vi "Periodic Tasks.vi"(8 "error in":errorcluster) -> ()   [LabVIEW 2016]
doc: "This VI runs in parallel to other tasks. It can contain as many user-defined periodic loops as you need. These can carry out PID or other sorts of timed response."
uses:
  Control 1.ctl
  <vilib>/Rock Robotics/WPI/Solenoid/WPI_SolenoidValue.ctl
  <vilib>/Rock Robotics/WPI/Utilities/WPI_GetSetVariantRefNum.vi
  <vilib>/Rock Robotics/WPI/Solenoid/WPI_SolenoidSetEnum.vi
  <vilib>/Rock Robotics/WPI/Solenoid/WPI_SolenoidGetEnum.vi
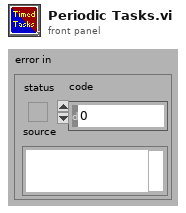
[diagram p1: front panel]
types:
  T1 = typedef "WPI_JoystickDevRef.ctl" = cluster{"Device":T2}
  T2 = typedef "WPI_JoystickDeviceEnum.ctl" = enum16{"USB 0", "USB 1", "USB 2", "USB 3", "USB 4", "USB 5"}
  T3 = typedef "Control 1.ctl" = enum16{"Off", "On"}
  T4 = typedef "WPI_SolenoidValue.ctl" = enum16{"Off", "On", "Forward", "Reverse"}
  T5 = typedef "WPI_SwitchDevRef.ctl" = cluster{"DevStatus":errorcluster, "DIO Channel":T6, "CntIndex":T7, "Normally Closed":bool}
  T6 = typedef "FPGA_DIOChannel.ctl" = enum8{"DIO 0", "DIO 1", "DIO 2", "DIO 3", "DIO 4", "DIO 5", "DIO 6", "DIO 7", "DIO 8", "DIO 9", "DIO MXP 0", "DIO MXP 1", "DIO MXP 2", "DIO MXP 3", "DIO MXP 4", "DIO MXP 5", "DIO MXP 6", "DIO MXP 7", "DIO MXP 8", "DIO MXP 9", "DIO MXP 10", "DIO MXP 11", "DIO MXP 12", "DIO MXP 13", "DIO MXP 14", "DIO MXP 15", "SPI Port CS1", "SPI Port CS2", "SPI Port CS3", "SPI Port MISO", "SPI Port MOSI", "Invalid"}
  T7 = typedef "FPGA_CounterCtrSystemIndex.ctl" = enum8{"Ctr 0", "Ctr 1", "Ctr 2", "Ctr 3", "Ctr 4", "Ctr 5", "Ctr 6", "Ctr 7", "Invalid"}
  T8 = typedef "WPI_SolenoidDevRef.ctl" = cluster{"DevStatus":errorcluster, "Pneumatics Control Module":u8, "Forward Solenoid Channel":T9, "Reverse Solenoid Channel":T9}
  T9 = typedef "WPI_SolenoidChannel.ctl" = enum8{"Solenoid 0", "Solenoid 1", "Solenoid 2", "Solenoid 3", "Solenoid 4", "Solenoid 5", "Solenoid 6", "Solenoid 7", "Invalid"}
  T10 = typedef "WPI_RelayDevRef.ctl" = cluster{"DevStatus":errorcluster, "Relay Channel":T11, "Relay Direction":T12}
  T11 = typedef "FPGA_DIORelayChannel.ctl" = enum8{"Relay 0", "Relay 1", "Relay 2", "Relay 3", "Invalid"}
  T12 = typedef "WPI_RelayDirection.ctl" = enum16{"Both directions", "Forward only", "Reverse only"}
  T13 = typedef "WPI_MotorControlDeviceRef.ctl" = cluster{"DeviceStatus":errorcluster, "Type":T14, "PWM":cluster{"PWM Channel":T15, "DeadBand":T16}, "CAN":cluster{"Device Number":u8, "SetOutput VI Ref":variant, "GetOutput VI Ref":variant, "Enable VI Ref":variant, "Disable VI Ref":variant, "Data":variant}, "Invert":bool}
  T14 = typedef "WPI_MotorControlType.ctl" = enum16{"PWM", "CAN"}
  T15 = typedef "FPGA_DIOPWMChannel.ctl" = enum8{"PWM 0", "PWM 1", "PWM 2", "PWM 3", "PWM 4", "PWM 5", "PWM 6", "PWM 7", "PWM 8", "PWM 9", "PWM MXP 0", "PWM MXP 1", "PWM MXP 2", "PWM MXP 3", "PWM MXP 4", "PWM MXP 5", "PWM MXP 6", "PWM MXP 7", "PWM MXP 8", "PWM MXP 9", "Invalid"}
  T16 = typedef "WPI_PWMDeadband.ctl" = cluster{"Name":string, "maxPositivePwm":i32, "minPositivePwm":i32, "centerPwm":i32, "maxNegativePwm":i32, "minNegativePwm":i32, "angularRange":u16}
  T17 = typedef "WPI_RobotDriveDevRef.ctl" = cluster{"DevStatus":errorcluster, "Motors[]":T13[], "Square Inputs":bool, "Max Output":dbl}
  T18 = cluster{"JoystickDevRef":T1, "JoystickDevRef":T1, "RobotDriveDevRef":T17}
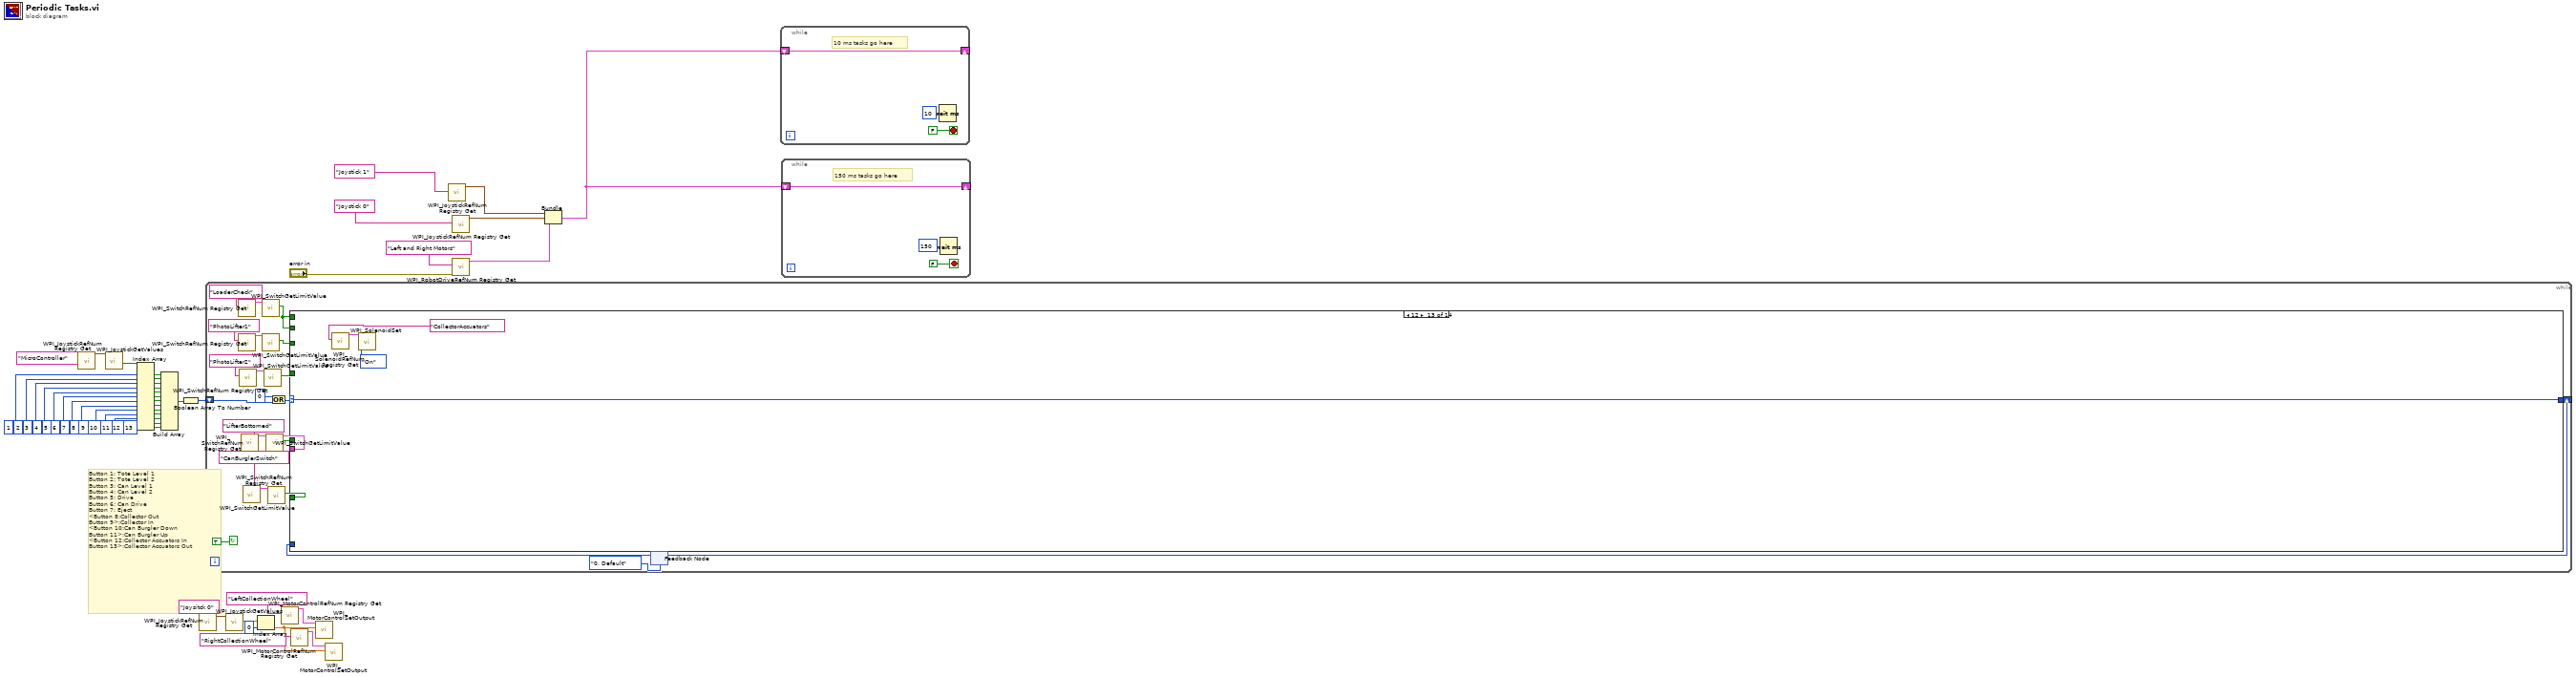
[diagram p0: block diagram]
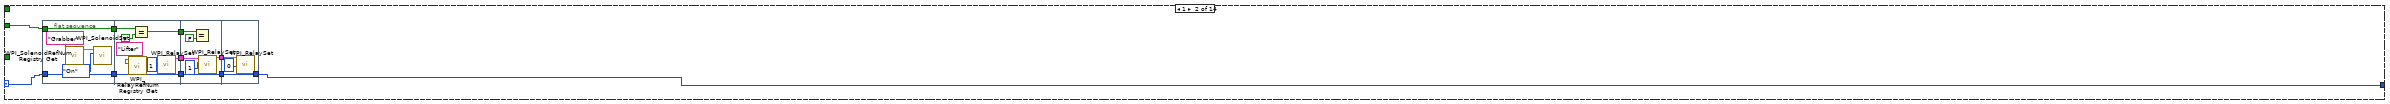
[diagram p3: hidden frame]
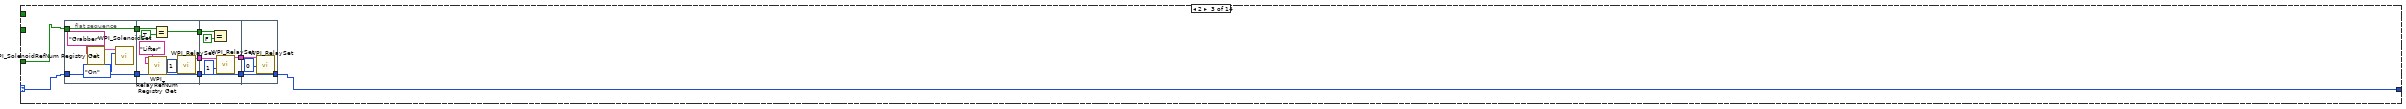
[diagram p4: hidden frame]
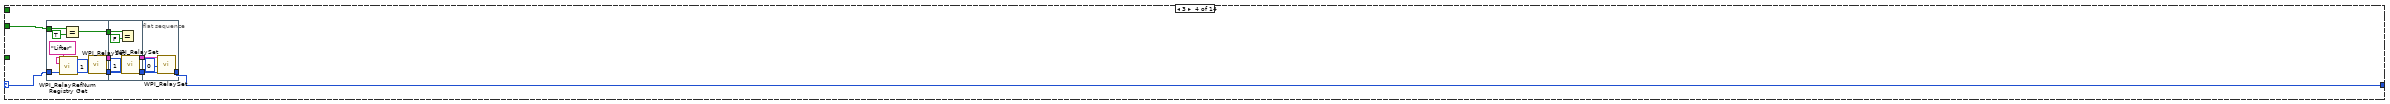
[diagram p5: hidden frame]
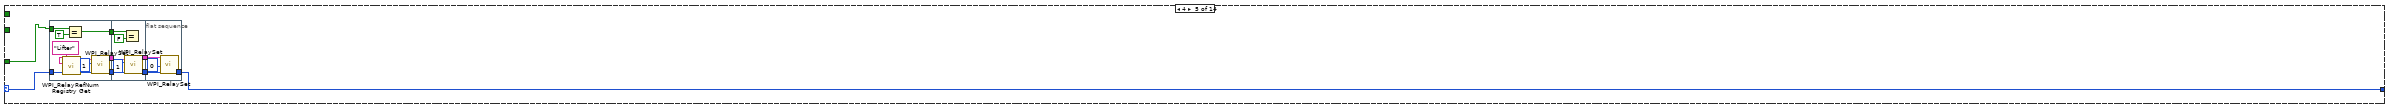
[diagram p6: hidden frame]
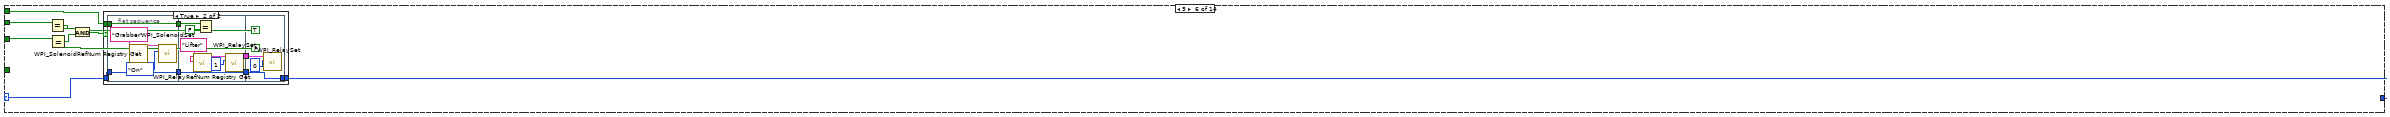
[diagram p7: hidden frame]
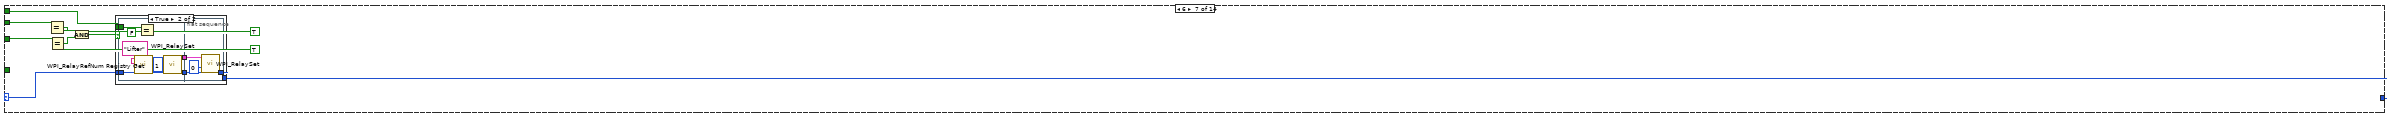
[diagram p9: hidden frame]
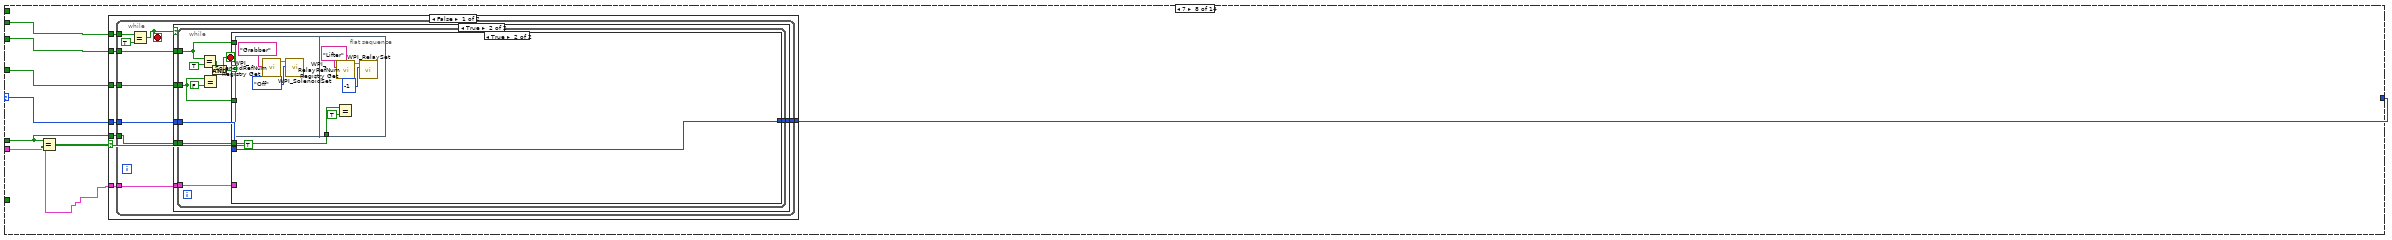
[diagram p11: hidden frame]
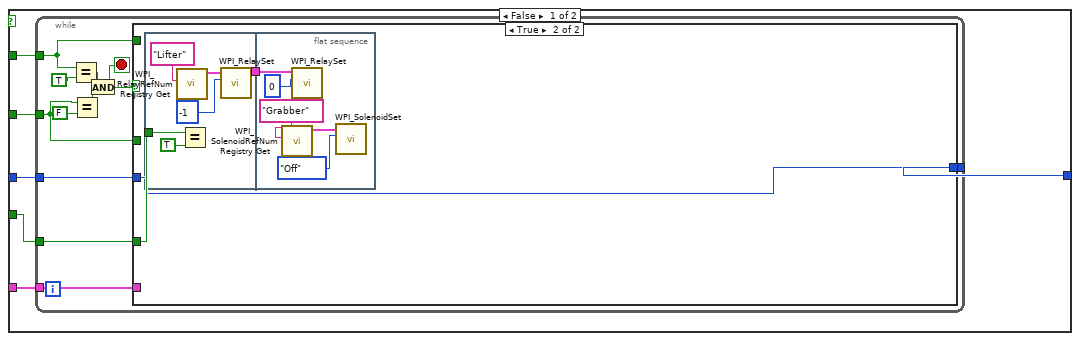
[diagram p12: hidden frame]
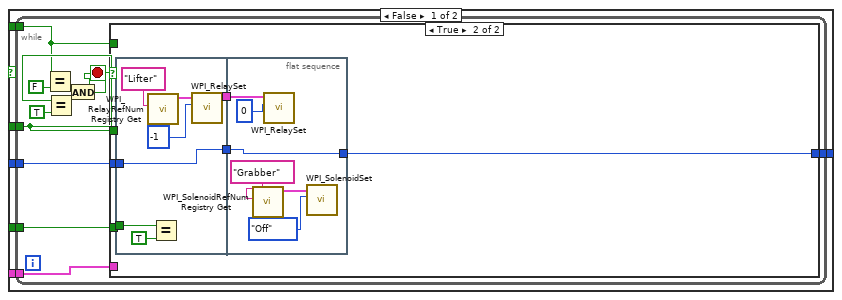
[diagram p13: hidden frame]
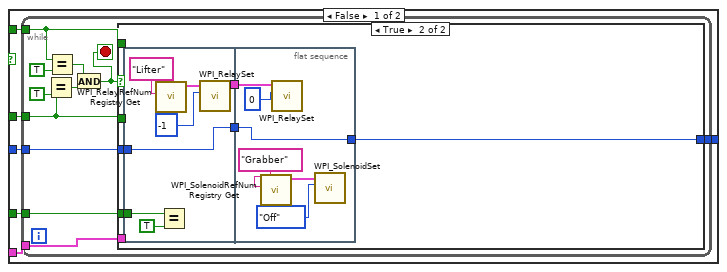
[diagram p14: hidden frame]
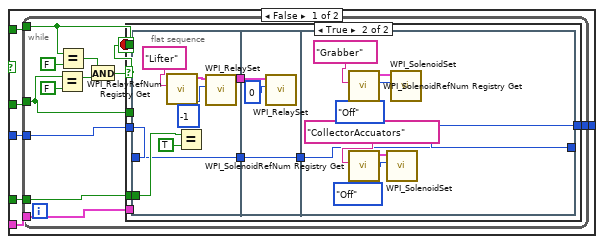
[diagram p15: hidden frame]
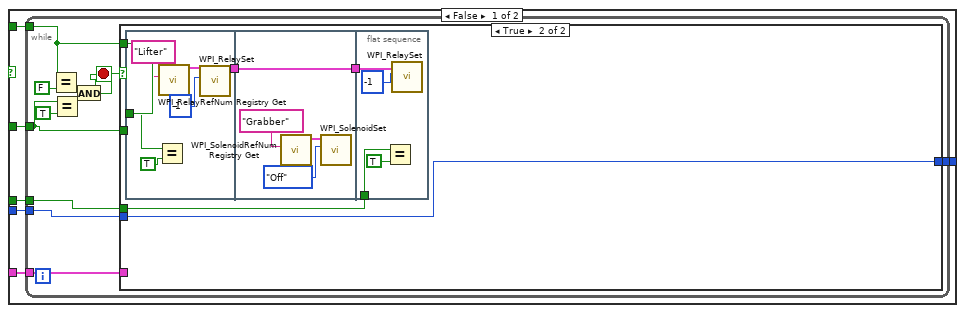
[diagram p17: hidden frame]
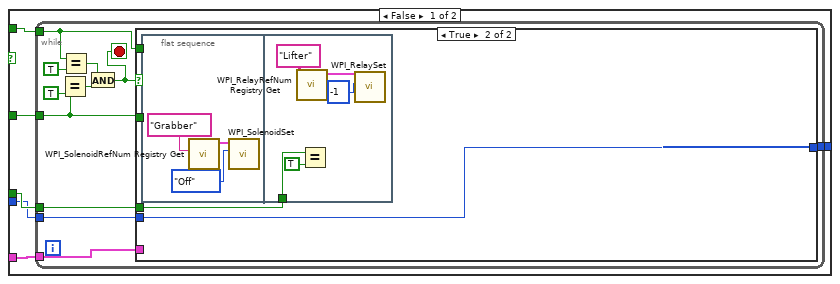
[diagram p18: hidden frame]
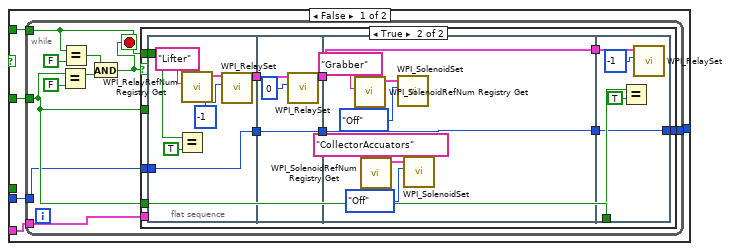
[diagram p19: hidden frame]
diagram:
  # "Button 1: Tote Level 1\nButton 2: Tote Level 2\nButton 3: Can Level 1\nButton 4: Can Level 2\nButton 5: Drive\nButton 6: Can Drive\nButton 7: Eject\n<Button 8:Collector Out\nButton 9>:Collector In\n<Button 10:Can Burgler Down\nButton 11>:Can Burgler Up\n<Button 12:Collector Accuators In\nButton 13>:Collector Accuators Out"
  n1 = call <vilib>:"WPI_JoystickRefNum Registry Get.vi"("refnum name"="MicroController") -> ("JoystickDevRef"=w40:T1)  [unwired: 9 in, 1 out]
  n2 = call <vilib>:"WPI_JoystickGetValues.vi"("JoystickDevRef"=w40) -> ("Buttons"=w39:bool[])  [unwired: 6 in, 4 out]
  n3 = Index Array(array=w39, index #1=1, index #2=2, index #3=3, index #4=4, index #5=5, index #6=6, index #7=7, index #8=8, index #9=9, index #10=10, index #11=11, index #12=12, index #13=13) -> (element #1=w25:bool, element #2=w24:bool, element #3=w23:bool, element #4=w22:bool, element #5=w21:bool, element #6=w20:bool, element #7=w19:bool, element #8=w18:bool, element #9=w17:bool, element #10=w16:bool, element #11=w15:bool, element #12=w14:bool, element #13=w13:bool)
  n4 = Build Array(w25, w24, w23, w22, w21, w20, w19, w18, w17, w16, w15, w14, w13) -> (w12:bool[])
  n5 = Boolean Array To Number(Boolean array=w12) -> (number=w11:u32)
  n6 = call <vilib>:"WPI_JoystickRefNum Registry Get.vi"("refnum name"="Joysitck 0") -> ("JoystickDevRef"=w9:T1)  [unwired: 9 in, 1 out]
  n7 = while {
    shift-right: [w58] -> _
    shift-left: w11 -> [w62]
    stop <- TRUE continue-if-true
    n8 = call <vilib>:"WPI_SwitchRefNum Registry Get.vi"("refnum name"="LoaderCheck") -> ("SwitchDevRef"=w65:T5)  [unwired: 9 in, 1 out]
    n9 = call <vilib>:"WPI_SwitchRefNum Registry Get.vi"("refnum name"="PhotoLifter1") -> ("SwitchDevRef"=w71:T5)  [unwired: 9 in, 1 out]
    n10 = call <vilib>:"WPI_SwitchRefNum Registry Get.vi"("refnum name"="PhotoLifter2") -> ("SwitchDevRef"=w70:T5)  [unwired: 9 in, 1 out]
    n11 = call <vilib>:"WPI_SwitchRefNum Registry Get.vi"("refnum name"="LifterBottomed") -> ("SwitchDevRef"=w55:T5)  [unwired: 9 in, 1 out]
    n12 = call <vilib>:"WPI_SwitchRefNum Registry Get.vi"("refnum name"="CanBurglerSwitch") -> ("SwitchDevRef"=w51:T5)  [unwired: 9 in, 1 out]
    n13 = call <vilib>:"WPI_SwitchGetLimitValue.vi"("SwitchDevRef"=w65) -> ("Switch Pressed"=w63:bool)  [unwired: 8 in, 2 out]
    n14 = call <vilib>:"WPI_SwitchGetLimitValue.vi"("SwitchDevRef"=w71) -> ("Switch Pressed"=w67:bool)  [unwired: 8 in, 2 out]
    n15 = call <vilib>:"WPI_SwitchGetLimitValue.vi"("SwitchDevRef"=w70) -> ("Switch Pressed"=w66:bool)  [unwired: 8 in, 2 out]
    n16 = call <vilib>:"WPI_SwitchGetLimitValue.vi"("SwitchDevRef"=w55) -> ("Switch Pressed"=w54:bool, "SwitchDevRef"=w52:T5)  [unwired: 8 in, 1 out]
    n17 = call <vilib>:"WPI_SwitchGetLimitValue.vi"("SwitchDevRef"=w51) -> ("Switch Pressed"=w49:bool)  [unwired: 8 in, 2 out]
    n18 = Or(x=0, y=w62) -> (x .or. y?=w60:u32)
    n19 = feedback #1(enum16{"0, Default"}."0, Default") -> (w57:u32)
    n20 = case shown="12" w60 {
      selector: w60 -> [w72 w76 w106 w138 w163 w189 w221 w247 w572 w580 _ _ w622 w626]
      tunnel: w67 -> [_ w82 _ w139 _ w196 w225 w251 _ _ _ _ _ _]
      tunnel: [w72 w75 w105 w137 w162 w187 w220 w246 w572 w579 _ _ w622 w626] -> w58
      tunnel: w66 -> [_ _ w107 _ w164 _ _ w250 _ _ _ _ _ _]
      tunnel: w63 -> [_ _ _ _ _ w194 w226 w252 _ w581 _ _ _ _]
      tunnel: w63 -> [_ _ _ _ _ w188 w222 _ _ _ _ _ _ _]
      tunnel: w57 -> [_ _ _ _ _ _ _ _ _ _ _ _ _ _]
      tunnel: w54 -> [_ _ _ _ _ _ _ w248 _ _ _ _ _ _]
      tunnel: w52 -> [_ _ _ _ _ _ _ w249 _ _ _ _ _ _]
      tunnel: w49 -> [_ _ _ _ _ _ _ _ _ _ _ w615 _ _]
      frame 0, Default {
      }
      frame 1 {
        n21 = flat-sequence {
          tunnel: w76 -> [w86]
          tunnel: w82 -> [w87]
          tunnel: [w87] -> w74
          tunnel: [w86] -> w73
          tunnel: [w90] -> w81
          tunnel: [w89] -> w80
          tunnel: [w88] -> w77
          tunnel: w74 -> [w93]
          tunnel: w73 -> [w88]
          tunnel: w81 -> [w101]
          tunnel: w80 -> [w99]
          tunnel: [w97] -> w79
          tunnel: [w96] -> w78
          tunnel: w77 -> [w96]
          tunnel: w79 -> [w104]
          tunnel: [w102] -> w75
          tunnel: w78 -> [w102]
          frame #0 {
            n22 = call <vilib>:"WPI_SolenoidRefNum Registry Get.vi"("refnum name"="Grabber") -> ("SolenoidDevRef"=w85:T8)  [unwired: 9 in, 1 out]
            n23 = call-poly <vilib>:"WPI_SolenoidSet.vi"("Value"=enum16{"Off", "On"}."On", "SolenoidDevRef"=w85) -> ()  [unwired: 8 in, 2 out]
          }
          frame #1 {
            n24 = call <vilib>:"WPI_RelayRefNum Registry Get.vi"("refnum name"="Lifter") -> ("RelayDevRef"=w95:T10)  [unwired: 9 in, 1 out]
            n25 = Equal?(x=w93, y=TRUE) -> (x = y?=w90:bool)
            n26 = call <vilib>:"WPI_RelaySet.vi"("RelayValue"=1, "RelayDevRef"=w95) -> ("RelayDevRef"=w89:T10)  [unwired: 8 in, 1 out]
          }
          frame #2 {
            n27 = Equal?(x=w101, y=FALSE) -> ()  [unwired: 1 out]
            n28 = call <vilib>:"WPI_RelaySet.vi"("RelayValue"=1, "RelayDevRef"=w99) -> ("RelayDevRef"=w97:T10)  [unwired: 8 in, 1 out]
          }
          frame #3 {
            n29 = call <vilib>:"WPI_RelaySet.vi"("RelayValue"=0, "RelayDevRef"=w104) -> ()  [unwired: 8 in, 2 out]
          }
        }
      }
      frame 2 {
        n30 = flat-sequence {
          tunnel: w106 -> [w118]
          tunnel: w107 -> [w119]
          tunnel: [w119] -> w114
          tunnel: [w118] -> w113
          tunnel: [w122] -> w112
          tunnel: [w121] -> w111
          tunnel: [w120] -> w110
          tunnel: w114 -> [w125]
          tunnel: w113 -> [w120]
          tunnel: w112 -> [w133]
          tunnel: w111 -> [w131]
          tunnel: [w129] -> w109
          tunnel: [w128] -> w108
          tunnel: w110 -> [w128]
          tunnel: w109 -> [w136]
          tunnel: [w134] -> w105
          tunnel: w108 -> [w134]
          frame #0 {
            n31 = call <vilib>:"WPI_SolenoidRefNum Registry Get.vi"("refnum name"="Grabber") -> ("SolenoidDevRef"=w117:T8)  [unwired: 9 in, 1 out]
            n32 = call-poly <vilib>:"WPI_SolenoidSet.vi"("Value"=enum16{"Off", "On"}."On", "SolenoidDevRef"=w117) -> ()  [unwired: 8 in, 2 out]
          }
          frame #1 {
            n33 = call <vilib>:"WPI_RelayRefNum Registry Get.vi"("refnum name"="Lifter") -> ("RelayDevRef"=w127:T10)  [unwired: 9 in, 1 out]
            n34 = Equal?(x=w125, y=TRUE) -> (x = y?=w122:bool)
            n35 = call <vilib>:"WPI_RelaySet.vi"("RelayValue"=1, "RelayDevRef"=w127) -> ("RelayDevRef"=w121:T10)  [unwired: 8 in, 1 out]
          }
          frame #2 {
            n36 = Equal?(x=w133, y=FALSE) -> ()  [unwired: 1 out]
            n37 = call <vilib>:"WPI_RelaySet.vi"("RelayValue"=1, "RelayDevRef"=w131) -> ("RelayDevRef"=w129:T10)  [unwired: 8 in, 1 out]
          }
          frame #3 {
            n38 = call <vilib>:"WPI_RelaySet.vi"("RelayValue"=0, "RelayDevRef"=w136) -> ()  [unwired: 8 in, 2 out]
          }
        }
      }
      frame 3 {
        n39 = flat-sequence {
          tunnel: [w147] -> w144
          tunnel: [w146] -> w143
          tunnel: [w145] -> w142
          tunnel: w139 -> [w150]
          tunnel: w138 -> [w145]
          tunnel: w144 -> [w158]
          tunnel: w143 -> [w156]
          tunnel: [w154] -> w141
          tunnel: [w153] -> w140
          tunnel: w142 -> [w153]
          tunnel: w141 -> [w161]
          tunnel: [w159] -> w137
          tunnel: w140 -> [w159]
          frame #0 {
            n40 = call <vilib>:"WPI_RelayRefNum Registry Get.vi"("refnum name"="Lifter") -> ("RelayDevRef"=w152:T10)  [unwired: 9 in, 1 out]
            n41 = Equal?(x=w150, y=TRUE) -> (x = y?=w147:bool)
            n42 = call <vilib>:"WPI_RelaySet.vi"("RelayValue"=1, "RelayDevRef"=w152) -> ("RelayDevRef"=w146:T10)  [unwired: 8 in, 1 out]
          }
          frame #1 {
            n43 = Equal?(x=w158, y=FALSE) -> ()  [unwired: 1 out]
            n44 = call <vilib>:"WPI_RelaySet.vi"("RelayValue"=1, "RelayDevRef"=w156) -> ("RelayDevRef"=w154:T10)  [unwired: 8 in, 1 out]
          }
          frame #2 {
            n45 = call <vilib>:"WPI_RelaySet.vi"("RelayValue"=0, "RelayDevRef"=w161) -> ()  [unwired: 8 in, 2 out]
          }
        }
      }
      frame 4 {
        n46 = flat-sequence {
          tunnel: [w172] -> w169
          tunnel: [w171] -> w168
          tunnel: [w170] -> w167
          tunnel: w164 -> [w175]
          tunnel: w163 -> [w170]
          tunnel: w169 -> [w183]
          tunnel: w168 -> [w181]
          tunnel: [w179] -> w166
          tunnel: [w178] -> w165
          tunnel: w167 -> [w178]
          tunnel: w166 -> [w186]
          tunnel: [w184] -> w162
          tunnel: w165 -> [w184]
          frame #0 {
            n47 = call <vilib>:"WPI_RelayRefNum Registry Get.vi"("refnum name"="Lifter") -> ("RelayDevRef"=w177:T10)  [unwired: 9 in, 1 out]
            n48 = Equal?(x=w175, y=TRUE) -> (x = y?=w172:bool)
            n49 = call <vilib>:"WPI_RelaySet.vi"("RelayValue"=1, "RelayDevRef"=w177) -> ("RelayDevRef"=w171:T10)  [unwired: 8 in, 1 out]
          }
          frame #1 {
            n50 = Equal?(x=w183, y=FALSE) -> ()  [unwired: 1 out]
            n51 = call <vilib>:"WPI_RelaySet.vi"("RelayValue"=1, "RelayDevRef"=w181) -> ("RelayDevRef"=w179:T10)  [unwired: 8 in, 1 out]
          }
          frame #2 {
            n52 = call <vilib>:"WPI_RelaySet.vi"("RelayValue"=0, "RelayDevRef"=w186) -> ()  [unwired: 8 in, 2 out]
          }
        }
      }
      frame 5 {
        n53 = Equal?(x=w194, y=TRUE) -> (x = y?=w192:bool)
        n54 = Equal?(x=w196, y=FALSE) -> (x = y?=w191:bool)
        n55 = And(x=w192, y=w191) -> (x .and. y?=w190:bool)
        n56 = case shown="True" w190 {
          tunnel: w189 -> [w197 w200]
          tunnel: w188 -> [_ w199]
          tunnel: [w197 w198] -> w187
          frame False {
          }
          frame True {
            n57 = flat-sequence {
              tunnel: w200 -> [w208]
              tunnel: w199 -> [w209]
              tunnel: [w209] -> w204
              tunnel: [w208] -> w203
              tunnel: [w211] -> w202
              tunnel: [w210] -> w201
              tunnel: w204 -> [w214]
              tunnel: w203 -> [w210]
              tunnel: w202 -> [w219]
              tunnel: w201 -> [w217]
              tunnel: [w217] -> w198
              frame #0 {
                n58 = call <vilib>:"WPI_SolenoidRefNum Registry Get.vi"("refnum name"="Grabber") -> ("SolenoidDevRef"=w207:T8)  [unwired: 9 in, 1 out]
                n59 = call-poly <vilib>:"WPI_SolenoidSet.vi"("Value"=enum16{"Off", "On"}."On", "SolenoidDevRef"=w207) -> ()  [unwired: 8 in, 2 out]
              }
              frame #1 {
                n60 = call <vilib>:"WPI_RelayRefNum Registry Get.vi"("refnum name"="Lifter") -> ("RelayDevRef"=w216:T10)  [unwired: 9 in, 1 out]
                n61 = Equal?(x=w214, y=FALSE) -> ()  [unwired: 1 out]
                n62 = call <vilib>:"WPI_RelaySet.vi"("RelayValue"=1, "RelayDevRef"=w216) -> ("RelayDevRef"=w211:T10)  [unwired: 8 in, 1 out]
              }
              frame #2 {
                n63 = call <vilib>:"WPI_RelaySet.vi"("RelayValue"=0, "RelayDevRef"=w219) -> ()  [unwired: 8 in, 2 out]
              }
            }
          }
        }
      }
      frame 6 {
        n64 = Equal?(x=w226, y=TRUE) -> (x = y?=w228:bool)
        n65 = Equal?(x=w225, y=TRUE) -> (x = y?=w227:bool)
        n66 = And(x=w228, y=w227) -> (x .and. y?=w223:bool)
        n67 = case shown="True" w223 {
          tunnel: w222 -> [_ w233]
          tunnel: w221 -> [w230 w232]
          tunnel: [w230 w231] -> w220
          frame False {
          }
          frame True {
            n68 = flat-sequence {
              tunnel: [w237] -> w235
              tunnel: [w236] -> w234
              tunnel: w233 -> [w240]
              tunnel: w232 -> [w236]
              tunnel: w235 -> [w245]
              tunnel: w234 -> [w243]
              tunnel: [w243] -> w231
              frame #0 {
                n69 = call <vilib>:"WPI_RelayRefNum Registry Get.vi"("refnum name"="Lifter") -> ("RelayDevRef"=w242:T10)  [unwired: 9 in, 1 out]
                n70 = Equal?(x=w240, y=FALSE) -> ()  [unwired: 1 out]
                n71 = call <vilib>:"WPI_RelaySet.vi"("RelayValue"=1, "RelayDevRef"=w242) -> ("RelayDevRef"=w237:T10)  [unwired: 8 in, 1 out]
              }
              frame #1 {
                n72 = call <vilib>:"WPI_RelaySet.vi"("RelayValue"=0, "RelayDevRef"=w245) -> ()  [unwired: 8 in, 2 out]
              }
            }
          }
        }
      }
      frame 7 {
        n73 = Equal?(x=w248, y=TRUE) -> (x = y?=w253:bool)
        n74 = case shown="False" w253 {
          tunnel: w252 -> [w261 _]
          tunnel: w251 -> [w260 _]
          tunnel: w250 -> [w259 _]
          tunnel: w249 -> [w258 _]
          tunnel: w248 -> [w257 _]
          tunnel: [w256 w553] -> w246
          tunnel: w247 -> [w255 w553]
          frame False {
            n75 = while {
              tunnel: w261 -> [w269]
              tunnel: w260 -> [w268]
              tunnel: w259 -> [w267]
              tunnel: w258 -> [w265]
              tunnel: w257 -> [w264]
              tunnel: [w263] -> w256
              tunnel: w255 -> [w262]
              stop <- w266 stop-if-true
              n76 = Equal?(x=w269, y=TRUE) -> (x = y?=w266:bool)
              n77 = case shown="True" w266 {
                tunnel: w268 -> [w276 w417]
                tunnel: w267 -> [w275 w416]
                tunnel: w265 -> [w274 w418]
                tunnel: w264 -> [w273 w415]
                tunnel: [w272 w414] -> w263
                tunnel: w262 -> [w271 w413]
                frame False {
                  n78 = while {
                    tunnel: w276 -> [w284]
                    tunnel: w275 -> [w283]
                    tunnel: w274 -> [w281]
                    tunnel: w273 -> [w279]
                    tunnel: [w278] -> w272
                    tunnel: w271 -> [w277]
                    stop <- w282 stop-if-true
                    n79 = Equal?(x=w284, y=TRUE) -> (x = y?=w286:bool)
                    n80 = Equal?(x=w283, y=FALSE) -> (x = y?=w285:bool)
                    n81 = And(x=w286, y=w285) -> (x .and. y?=w282:bool)
                    n82 = case shown="True" w282 {
                      tunnel: w284 -> [w293 _]
                      tunnel: w283 -> [w292 _]
                      tunnel: w281 -> [w291 _]
                      tunnel: w279 -> [w290 w400]
                      tunnel: [w288 w399] -> w278
                      tunnel: w277 -> [w289 w399]
                      frame False {
                        n83 = while {
                          tunnel: w293 -> [w299]
                          tunnel: w292 -> [w300]
                          tunnel: w291 -> [w297]
                          tunnel: w290 -> [w296]
                          tunnel: w289 -> [w295]
                          tunnel: [w294] -> w288
                          stop <- w298 stop-if-true
                          n84 = Equal?(x=w299, y=FALSE) -> (x = y?=w304:bool)
                          n85 = Equal?(x=w300, y=TRUE) -> (x = y?=w303:bool)
                          n86 = And(x=w304, y=w303) -> (x .and. y?=w298:bool)
                          n87 = case shown="True" w298 {
                            tunnel: w300 -> [w310 _]
                            tunnel: w299 -> [w309 _]
                            tunnel: w297 -> [w308 _]
                            tunnel: w296 -> [w307 w384]
                            tunnel: w295 -> [w306 w382]
                            tunnel: [w305 w381] -> w294
                            frame False {
                              n88 = while {
                                tunnel: w310 -> [w316]
                                tunnel: w309 -> [w315]
                                tunnel: w308 -> [w314]
                                tunnel: w307 -> [w313]
                                tunnel: w306 -> [w312]
                                tunnel: [w311] -> w305
                                stop <- w317 stop-if-true
                                n89 = Equal?(x=w316, y=TRUE) -> (x = y?=w320:bool)
                                n90 = Equal?(x=w315, y=TRUE) -> (x = y?=w321:bool)
                                n91 = And(x=w321, y=w320) -> (x .and. y?=w317:bool)
                                n92 = case shown="True" w317 {
                                tunnel: w316 -> [w326 _]
                                tunnel: w315 -> [w327 _]
                                tunnel: w314 -> [w325 _]
                                tunnel: w313 -> [w324 w367]
                                tunnel: w312 -> [w323 w364]
                                tunnel: [w322 w363] -> w311
                                frame False {
                                n93 = while {
                                tunnel: w327 -> [w333]
                                tunnel: w326 -> [w331]
                                tunnel: w325 -> [w332]
                                tunnel: w324 -> [w330]
                                tunnel: w323 -> [w329]
                                tunnel: [w328] -> w322
                                stop <- w334 stop-if-true
                                n94 = Equal?(x=w331, y=FALSE) -> (x = y?=w336:bool)
                                n95 = Equal?(x=w333, y=FALSE) -> (x = y?=w335:bool)
                                n96 = And(x=w335, y=w336) -> (x .and. y?=w334:bool)
                                n97 = case shown="True" w334 {
                                tunnel: w333 -> [_ _]
                                tunnel: w331 -> [_ _]
                                tunnel: w332 -> [_ _]
                                tunnel: w330 -> [_ w345]
                                tunnel: w329 -> [w339 w342]
                                tunnel: [w339 w340] -> w328
                                frame False {
                                }
                                frame True {
                                n98 = flat-sequence {
                                tunnel: w345 -> [w348]
                                tunnel: [w347] -> w344
                                tunnel: [w346] -> w343
                                tunnel: w342 -> [w346]
                                tunnel: w344 -> [w355]
                                tunnel: w343 -> [w353]
                                tunnel: [w353] -> w341
                                tunnel: w341 -> [w356]
                                tunnel: [w356] -> w340
                                frame #0 {
                                n99 = call <vilib>:"WPI_RelayRefNum Registry Get.vi"("refnum name"="Lifter") -> ("RelayDevRef"=w352:T10)  [unwired: 9 in, 1 out]
                                n100 = Equal?(x=w348, y=TRUE) -> ()  [unwired: 1 out]
                                n101 = call <vilib>:"WPI_RelaySet.vi"("RelayValue"=-1, "RelayDevRef"=w352) -> ("RelayDevRef"=w347:T10)  [unwired: 8 in, 1 out]
                                }
                                frame #1 {
                                n102 = call <vilib>:"WPI_RelaySet.vi"("RelayValue"=0, "RelayDevRef"=w355) -> ()  [unwired: 8 in, 2 out]
                                }
                                frame #2 {
                                n103 = call <vilib>:"WPI_SolenoidRefNum Registry Get.vi"("refnum name"="Grabber") -> ("SolenoidDevRef"=w362:T8)  [unwired: 9 in, 1 out]
                                n104 = call <vilib>:"WPI_SolenoidRefNum Registry Get.vi"("refnum name"="CollectorAccuators") -> ("SolenoidDevRef"=w360:T8)  [unwired: 9 in, 1 out]
                                n105 = call-poly <vilib>:"WPI_SolenoidSet.vi"("Value"=enum16{"Off", "On"}."Off", "SolenoidDevRef"=w360) -> ()  [unwired: 8 in, 2 out]
                                n106 = call-poly <vilib>:"WPI_SolenoidSet.vi"("Value"=enum16{"Off", "On"}."Off", "SolenoidDevRef"=w362) -> ()  [unwired: 8 in, 2 out]
                                }
                                }
                                }
                                }
                                }
                                }
                                frame True {
                                n107 = flat-sequence {
                                tunnel: w367 -> [w371]
                                tunnel: [w369] -> w366
                                tunnel: [w368] -> w365
                                tunnel: w364 -> [w368]
                                tunnel: w366 -> [w380]
                                tunnel: w365 -> [w375]
                                tunnel: [w375] -> w363
                                frame #0 {
                                n108 = call <vilib>:"WPI_RelayRefNum Registry Get.vi"("refnum name"="Lifter") -> ("RelayDevRef"=w374:T10)  [unwired: 9 in, 1 out]
                                n109 = Equal?(x=w371, y=TRUE) -> ()  [unwired: 1 out]
                                n110 = call <vilib>:"WPI_RelaySet.vi"("RelayValue"=-1, "RelayDevRef"=w374) -> ("RelayDevRef"=w369:T10)  [unwired: 8 in, 1 out]
                                }
                                frame #1 {
                                n111 = call <vilib>:"WPI_SolenoidRefNum Registry Get.vi"("refnum name"="Grabber") -> ("SolenoidDevRef"=w378:T8)  [unwired: 9 in, 1 out]
                                n112 = call <vilib>:"WPI_RelaySet.vi"("RelayValue"=0, "RelayDevRef"=w380) -> ()  [unwired: 8 in, 2 out]
                                n113 = call-poly <vilib>:"WPI_SolenoidSet.vi"("Value"=enum16{"Off", "On"}."Off", "SolenoidDevRef"=w378) -> ()  [unwired: 8 in, 2 out]
                                }
                                }
                                }
                                }
                              }
                            }
                            frame True {
                              n114 = flat-sequence {
                                tunnel: w384 -> [w389]
                                tunnel: [w387] -> w385
                                tunnel: [w386] -> w383
                                tunnel: w382 -> [w386]
                                tunnel: w385 -> [w398]
                                tunnel: w383 -> [w393]
                                tunnel: [w393] -> w381
                                frame #0 {
                                n115 = call <vilib>:"WPI_RelayRefNum Registry Get.vi"("refnum name"="Lifter") -> ("RelayDevRef"=w392:T10)  [unwired: 9 in, 1 out]
                                n116 = Equal?(x=w389, y=TRUE) -> ()  [unwired: 1 out]
                                n117 = call <vilib>:"WPI_RelaySet.vi"("RelayValue"=-1, "RelayDevRef"=w392) -> ("RelayDevRef"=w387:T10)  [unwired: 8 in, 1 out]
                                }
                                frame #1 {
                                n118 = call <vilib>:"WPI_SolenoidRefNum Registry Get.vi"("refnum name"="Grabber") -> ("SolenoidDevRef"=w396:T8)  [unwired: 9 in, 1 out]
                                n119 = call <vilib>:"WPI_RelaySet.vi"("RelayValue"=0, "RelayDevRef"=w398) -> ()  [unwired: 8 in, 2 out]
                                n120 = call-poly <vilib>:"WPI_SolenoidSet.vi"("Value"=enum16{"Off", "On"}."Off", "SolenoidDevRef"=w396) -> ()  [unwired: 8 in, 2 out]
                                }
                              }
                            }
                          }
                        }
                      }
                      frame True {
                        n121 = flat-sequence {
                          tunnel: w400 -> [w404]
                          tunnel: [w402] -> w401
                          tunnel: w401 -> [w412]
                          frame #0 {
                            n122 = call <vilib>:"WPI_RelayRefNum Registry Get.vi"("refnum name"="Lifter") -> ("RelayDevRef"=w407:T10)  [unwired: 9 in, 1 out]
                            n123 = Equal?(x=w404, y=TRUE) -> ()  [unwired: 1 out]
                            n124 = call <vilib>:"WPI_RelaySet.vi"("RelayValue"=-1, "RelayDevRef"=w407) -> ("RelayDevRef"=w402:T10)  [unwired: 8 in, 1 out]
                          }
                          frame #1 {
                            n125 = call <vilib>:"WPI_SolenoidRefNum Registry Get.vi"("refnum name"="Grabber") -> ("SolenoidDevRef"=w410:T8)  [unwired: 9 in, 1 out]
                            n126 = call <vilib>:"WPI_RelaySet.vi"("RelayValue"=0, "RelayDevRef"=w412) -> ()  [unwired: 8 in, 2 out]
                            n127 = call-poly <vilib>:"WPI_SolenoidSet.vi"("Value"=enum16{"Off", "On"}."Off", "SolenoidDevRef"=w410) -> ()  [unwired: 8 in, 2 out]
                          }
                        }
                      }
                    }
                  }
                }
                frame True {
                  n128 = while {
                    tunnel: w417 -> [w426]
                    tunnel: w416 -> [w425]
                    tunnel: w418 -> [w423]
                    tunnel: w415 -> [w421]
                    tunnel: [w420] -> w414
                    tunnel: w413 -> [w419]
                    stop <- w424 stop-if-true
                    n129 = Equal?(x=w426, y=TRUE) -> (x = y?=w428:bool)
                    n130 = Equal?(x=w425, y=FALSE) -> (x = y?=w427:bool)
                    n131 = And(x=w428, y=w427) -> (x .and. y?=w424:bool)
                    n132 = case shown="True" w424 {
                      tunnel: w426 -> [w435 _]
                      tunnel: w425 -> [w434 _]
                      tunnel: w423 -> [w433 _]
                      tunnel: w421 -> [w432 w544]
                      tunnel: [w430 w543] -> w420
                      tunnel: w419 -> [w431 w543]
                      frame False {
                        n133 = while {
                          tunnel: w435 -> [w441]
                          tunnel: w434 -> [w442]
                          tunnel: w433 -> [w439]
                          tunnel: w432 -> [w438]
                          tunnel: w431 -> [w437]
                          tunnel: [w436] -> w430
                          stop <- w440 stop-if-true
                          n134 = Equal?(x=w441, y=FALSE) -> (x = y?=w446:bool)
                          n135 = Equal?(x=w442, y=TRUE) -> (x = y?=w445:bool)
                          n136 = And(x=w446, y=w445) -> (x .and. y?=w440:bool)
                          n137 = case shown="True" w440 {
                            tunnel: w442 -> [w452 _]
                            tunnel: w441 -> [w451 w527]
                            tunnel: w439 -> [w450 _]
                            tunnel: w438 -> [w449 w528]
                            tunnel: w437 -> [w447 w524]
                            tunnel: [w448 w524] -> w436
                            frame False {
                              n138 = while {
                                tunnel: w452 -> [w458]
                                tunnel: w451 -> [w457]
                                tunnel: w450 -> [w456]
                                tunnel: w449 -> [w455]
                                tunnel: [w454] -> w448
                                tunnel: w447 -> [w453]
                                stop <- w459 stop-if-true
                                n139 = Equal?(x=w458, y=TRUE) -> (x = y?=w462:bool)
                                n140 = Equal?(x=w457, y=TRUE) -> (x = y?=w463:bool)
                                n141 = And(x=w463, y=w462) -> (x .and. y?=w459:bool)
                                n142 = case shown="True" w459 {
                                tunnel: w458 -> [w467 _]
                                tunnel: w457 -> [w468 _]
                                tunnel: w456 -> [w466 _]
                                tunnel: w455 -> [_ w515]
                                tunnel: [w464 w514] -> w454
                                tunnel: w453 -> [w465 w514]
                                frame False {
                                n143 = while {
                                tunnel: w468 -> [w473]
                                tunnel: w467 -> [w471]
                                tunnel: w466 -> [w472]
                                tunnel: w465 -> [w470]
                                tunnel: [w469] -> w464
                                stop <- w474 stop-if-true
                                n144 = Equal?(x=w471, y=FALSE) -> (x = y?=w476:bool)
                                n145 = Equal?(x=w473, y=FALSE) -> (x = y?=w475:bool)
                                n146 = And(x=w475, y=w476) -> (x .and. y?=w474:bool)
                                n147 = case shown="True" w474 {
                                tunnel: w473 -> [_ w489]
                                tunnel: w471 -> [_ _]
                                tunnel: w472 -> [_ _]
                                tunnel: w471 -> [_ w485]
                                tunnel: w470 -> [w479 w482]
                                tunnel: [w479 w480] -> w469
                                frame False {
                                }
                                frame True {
                                n148 = flat-sequence {
                                tunnel: w489 -> [w493]
                                tunnel: [w491] -> w488
                                tunnel: [w490] -> w483
                                tunnel: w482 -> [w490]
                                tunnel: w488 -> [w500]
                                tunnel: [w498] -> w486
                                tunnel: [w497] -> w484
                                tunnel: w483 -> [w497]
                                tunnel: [w502] -> w487
                                tunnel: w486 -> [w502]
                                tunnel: w484 -> [w501]
                                tunnel: [w501] -> w481
                                tunnel: w487 -> [w513]
                                tunnel: w485 -> [w511]
                                tunnel: w481 -> [w509]
                                tunnel: [w509] -> w480
                                frame #0 {
                                n149 = Equal?(x=w493, y=TRUE) -> ()  [unwired: 1 out]
                                n150 = call <vilib>:"WPI_RelayRefNum Registry Get.vi"("refnum name"="Lifter") -> ("RelayDevRef"=w496:T10)  [unwired: 9 in, 1 out]
                                n151 = call <vilib>:"WPI_RelaySet.vi"("RelayValue"=-1, "RelayDevRef"=w496) -> ("RelayDevRef"=w491:T10)  [unwired: 8 in, 1 out]
                                }
                                frame #1 {
                                n152 = call <vilib>:"WPI_RelaySet.vi"("RelayValue"=0, "RelayDevRef"=w500) -> ("RelayDevRef"=w498:T10)  [unwired: 8 in, 1 out]
                                }
                                frame #2 {
                                n153 = call <vilib>:"WPI_SolenoidRefNum Registry Get.vi"("refnum name"="Grabber") -> ("SolenoidDevRef"=w508:T8)  [unwired: 9 in, 1 out]
                                n154 = call <vilib>:"WPI_SolenoidRefNum Registry Get.vi"("refnum name"="CollectorAccuators") -> ("SolenoidDevRef"=w505:T8)  [unwired: 9 in, 1 out]
                                n155 = call-poly <vilib>:"WPI_SolenoidSet.vi"("Value"=enum16{"Off", "On"}."Off", "SolenoidDevRef"=w508) -> ()  [unwired: 8 in, 2 out]
                                n156 = call-poly <vilib>:"WPI_SolenoidSet.vi"("Value"=enum16{"Off", "On"}."Off", "SolenoidDevRef"=w505) -> ()  [unwired: 8 in, 2 out]
                                }
                                frame #3 {
                                n157 = Equal?(x=w511, y=TRUE) -> ()  [unwired: 1 out]
                                n158 = call <vilib>:"WPI_RelaySet.vi"("RelayValue"=-1, "RelayDevRef"=w513) -> ()  [unwired: 8 in, 2 out]
                                }
                                }
                                }
                                }
                                }
                                }
                                frame True {
                                n159 = flat-sequence {
                                tunnel: w515 -> [w522]
                                frame #0 {
                                n160 = call <vilib>:"WPI_SolenoidRefNum Registry Get.vi"("refnum name"="Grabber") -> ("SolenoidDevRef"=w518:T8)  [unwired: 9 in, 1 out]
                                n161 = call-poly <vilib>:"WPI_SolenoidSet.vi"("Value"=enum16{"Off", "On"}."Off", "SolenoidDevRef"=w518) -> ()  [unwired: 8 in, 2 out]
                                }
                                frame #1 {
                                n162 = call <vilib>:"WPI_RelayRefNum Registry Get.vi"("refnum name"="Lifter") -> ("RelayDevRef"=w520:T10)  [unwired: 9 in, 1 out]
                                n163 = Equal?(x=w522, y=TRUE) -> ()  [unwired: 1 out]
                                n164 = call <vilib>:"WPI_RelaySet.vi"("RelayValue"=-1, "RelayDevRef"=w520) -> ()  [unwired: 8 in, 2 out]
                                }
                                }
                                }
                                }
                              }
                            }
                            frame True {
                              n165 = flat-sequence {
                                tunnel: w527 -> [w530]
                                tunnel: [w529] -> w525
                                tunnel: [w535] -> w526
                                tunnel: w525 -> [w535]
                                tunnel: w528 -> [w541]
                                tunnel: w526 -> [w539]
                                frame #0 {
                                n166 = Equal?(x=w530, y=TRUE) -> ()  [unwired: 1 out]
                                n167 = call <vilib>:"WPI_RelayRefNum Registry Get.vi"("refnum name"="Lifter") -> ("RelayDevRef"=w533:T10)  [unwired: 9 in, 1 out]
                                n168 = call <vilib>:"WPI_RelaySet.vi"("RelayValue"=-1, "RelayDevRef"=w533) -> ("RelayDevRef"=w529:T10)  [unwired: 8 in, 1 out]
                                }
                                frame #1 {
                                n169 = call <vilib>:"WPI_SolenoidRefNum Registry Get.vi"("refnum name"="Grabber") -> ("SolenoidDevRef"=w538:T8)  [unwired: 9 in, 1 out]
                                n170 = call-poly <vilib>:"WPI_SolenoidSet.vi"("Value"=enum16{"Off", "On"}."Off", "SolenoidDevRef"=w538) -> ()  [unwired: 8 in, 2 out]
                                }
                                frame #2 {
                                n171 = Equal?(x=w541, y=TRUE) -> ()  [unwired: 1 out]
                                n172 = call <vilib>:"WPI_RelaySet.vi"("RelayValue"=-1, "RelayDevRef"=w539) -> ()  [unwired: 8 in, 2 out]
                                }
                              }
                            }
                          }
                        }
                      }
                      frame True {
                        n173 = flat-sequence {
                          tunnel: w544 -> [w549]
                          frame #0 {
                            n174 = call <vilib>:"WPI_SolenoidRefNum Registry Get.vi"("refnum name"="Grabber") -> ("SolenoidDevRef"=w547:T8)  [unwired: 9 in, 1 out]
                            n175 = call-poly <vilib>:"WPI_SolenoidSet.vi"("Value"=enum16{"Off", "On"}."Off", "SolenoidDevRef"=w547) -> ()  [unwired: 8 in, 2 out]
                          }
                          frame #1 {
                            n176 = Equal?(x=w549, y=TRUE) -> ()  [unwired: 1 out]
                            n177 = call <vilib>:"WPI_RelayRefNum Registry Get.vi"("refnum name"="Lifter") -> ("RelayDevRef"=w552:T10)  [unwired: 9 in, 1 out]
                            n178 = call <vilib>:"WPI_RelaySet.vi"("RelayValue"=-1, "RelayDevRef"=w552) -> ()  [unwired: 8 in, 2 out]
                          }
                        }
                      }
                    }
                  }
                }
              }
            }
          }
          frame True {
            n179 = while {
              stop <- w554 stop-if-true
              n180 = call <vilib>:"WPI_SolenoidRefNum Registry Get.vi"("refnum name"="Grabber") -> ("SolenoidDevRef"=w560:T8)  [unwired: 9 in, 1 out]
              n181 = call-poly <vilib>:"WPI_SolenoidGet.vi"("SolenoidDevRef"=w560) -> ("Value"=w558:T4, "SolenoidDevRef"=w557:T8)  [unwired: 8 in, 1 out]
              n182 = Equal?(x=w558, y=Control_1."On") -> (x = y?=w554:bool)
              n183 = call <vilib>:"WPI_SolenoidRefNum Registry Get.vi"("refnum name"="CollectorAccuators") -> ("SolenoidDevRef"=w555:T8)  [unwired: 9 in, 1 out]
              n184 = case shown="True" w554 {
                tunnel: w557 -> [_ w566]
                tunnel: w555 -> [w563 w565]
                frame False {
                  n185 = call-poly <vilib>:"WPI_SolenoidSet.vi"("Value"=Control_1."Off", "SolenoidDevRef"=w563) -> ()  [unwired: 8 in, 2 out]
                }
                frame True {
                  n186 = flat-sequence {
                    tunnel: w566 -> [w569]
                    tunnel: w565 -> [w567]
                    tunnel: [w567] -> w564
                    tunnel: w564 -> [w571]
                    frame #0 {
                      n187 = call-poly <vilib>:"WPI_SolenoidSet.vi"("Value"=Control_1."Off", "SolenoidDevRef"=w569) -> ()  [unwired: 8 in, 2 out]
                    }
                    frame #1 {
                      n188 = call-poly <vilib>:"WPI_SolenoidSet.vi"("Value"=Control_1."Off", "SolenoidDevRef"=w571) -> ()  [unwired: 8 in, 2 out]
                    }
                  }
                }
              }
            }
          }
        }
      }
      frame 8 {
        n189 = call <vilib>:"WPI_MotorControlRefNum Registry Get.vi"("refnum name"="LeftCollectionWheel") -> ("MotorControlDevRef"=w578:T13)  [unwired: 9 in, 1 out]
        n190 = call <vilib>:"WPI_MotorControlRefNum Registry Get.vi"("refnum name"="RightCollectionWheel") -> ("MotorControlDevRef"=w576:T13)  [unwired: 9 in, 1 out]
        n191 = call <vilib>:"WPI_MotorControlSetOutput.vi"("Output"=1.0, "MotorControlDevRef"=w578) -> ()  [unwired: 7 in, 3 out]
        n192 = call <vilib>:"WPI_MotorControlSetOutput.vi"("Output"=1.0, "MotorControlDevRef"=w576) -> ()  [unwired: 7 in, 3 out]
      }
      frame 9 {
        n193 = while {
          tunnel: w581 -> [w585]
          tunnel: w580 -> [w583]
          tunnel: [w582] -> w579
          stop <- w584 stop-if-true
          n194 = call <vilib>:"WPI_MotorControlRefNum Registry Get.vi"("refnum name"="LeftCollectionWheel") -> ("MotorControlDevRef"=w595:T13)  [unwired: 9 in, 1 out]
          n195 = call <vilib>:"WPI_MotorControlRefNum Registry Get.vi"("refnum name"="RightCollectionWheel") -> ("MotorControlDevRef"=w593:T13)  [unwired: 9 in, 1 out]
          n196 = call <vilib>:"WPI_MotorControlSetOutput.vi"("Output"=-1.0, "MotorControlDevRef"=w595) -> ("MotorControlDevRef"=w587:T13)  [unwired: 7 in, 2 out]
          n197 = call <vilib>:"WPI_MotorControlSetOutput.vi"("Output"=-1.0, "MotorControlDevRef"=w593) -> ("MotorControlDevRef"=w586:T13)  [unwired: 7 in, 2 out]
          n198 = Equal?(x=w585, y=FALSE) -> (x = y?=w588:bool)
          n199 = case shown="True" w588 {
            selector: w588 -> [_ w602]
            tunnel: w587 -> [w598 w606]
            tunnel: w586 -> [w597 w605]
            tunnel: [_ w602] -> w584
            tunnel: w583 -> [w596 w601]
            tunnel: [w596 w601] -> w582
            frame False {
              n200 = call <vilib>:"WPI_MotorControlSetOutput.vi"("Output"=-1.0, "MotorControlDevRef"=w597) -> ()  [unwired: 7 in, 3 out]
              n201 = call <vilib>:"WPI_MotorControlSetOutput.vi"("Output"=-1.0, "MotorControlDevRef"=w598) -> ()  [unwired: 7 in, 3 out]
            }
            frame True {
              n202 = call <vilib>:"WPI_MotorControlSetOutput.vi"("Output"=0.0, "MotorControlDevRef"=w605) -> ()  [unwired: 7 in, 3 out]
              n203 = call <vilib>:"WPI_MotorControlSetOutput.vi"("Output"=0.0, "MotorControlDevRef"=w606) -> ()  [unwired: 7 in, 3 out]
            }
          }
        }
      }
      frame 10 {
        n204 = call <vilib>:"WPI_MotorControlRefNum Registry Get.vi"("refnum name"="CanBurglers") -> ("MotorControlDevRef"=w609:T13)  [unwired: 9 in, 1 out]
        n205 = call <vilib>:"WPI_MotorControlSetOutput.vi"("Output"=1.0, "MotorControlDevRef"=w609) -> ()  [unwired: 7 in, 3 out]
      }
      frame 11 {
        n206 = call <vilib>:"WPI_MotorControlRefNum Registry Get.vi"("refnum name"="CanBurgler") -> ("MotorControlDevRef"=w613:T13)  [unwired: 9 in, 1 out]
        n207 = Equal?(x=w615, y=TRUE) -> (x = y?=w614:bool)
        n208 = call <vilib>:"WPI_MotorControlSetOutput.vi"("Output"=-1.0, "MotorControlDevRef"=w613) -> ("MotorControlDevRef"=w610:T13)  [unwired: 7 in, 2 out]
        n209 = case shown="True" w614 {
          tunnel: w610 -> [w618 w620]
          frame False {
            n210 = call <vilib>:"WPI_MotorControlSetOutput.vi"("Output"=-1.0, "MotorControlDevRef"=w618) -> ()  [unwired: 7 in, 3 out]
          }
          frame True {
            n211 = call <vilib>:"WPI_MotorControlSetOutput.vi"("Output"=0.0, "MotorControlDevRef"=w620) -> ()  [unwired: 7 in, 3 out]
          }
        }
      }
      frame 12 {
        n212 = call <vilib>:"WPI_SolenoidRefNum Registry Get.vi"("refnum name"="CollectorAccuators") -> ("SolenoidDevRef"=w624:T8)  [unwired: 9 in, 1 out]
        n213 = call-poly <vilib>:"WPI_SolenoidSet.vi"("Value"=WPI_SolenoidValue."On", "SolenoidDevRef"=w624) -> ()  [unwired: 8 in, 2 out]
      }
      frame 13 {
        n214 = call <vilib>:"WPI_SolenoidRefNum Registry Get.vi"("refnum name"="CollectorAccuators") -> ("SolenoidDevRef"=w628:T8)  [unwired: 9 in, 1 out]
        n215 = call-poly <vilib>:"WPI_SolenoidSet.vi"("Value"=WPI_SolenoidValue."Off", "SolenoidDevRef"=w628) -> ()  [unwired: 8 in, 2 out]
      }
    }
    n216 = feedback-in #1(w58) -> ()
  }
  n217 = call <vilib>:"WPI_JoystickGetValues.vi"("JoystickDevRef"=w9) -> ("Axes"=w7:dbl[])  [unwired: 6 in, 4 out]
  n218 = Index Array(array=w7, index=0) -> (element=w3:dbl)
  n219 = call <vilib>:"WPI_MotorControlRefNum Registry Get.vi"("refnum name"="LeftCollectionWheel") -> ("MotorControlDevRef"=w5:T13)  [unwired: 9 in, 1 out]
  n220 = call <vilib>:"WPI_MotorControlRefNum Registry Get.vi"("refnum name"="RightCollectionWheel") -> ("MotorControlDevRef"=w4:T13)  [unwired: 9 in, 1 out]
  n221 = call <vilib>:"WPI_MotorControlSetOutput.vi"("Output"=w3, "MotorControlDevRef"=w5) -> ()  [unwired: 7 in, 3 out]
  n222 = call <vilib>:"WPI_MotorControlSetOutput.vi"("Output"=w3, "MotorControlDevRef"=w4) -> ()  [unwired: 7 in, 3 out]
  n223 = call <vilib>:"WPI_JoystickRefNum Registry Get.vi"("refnum name"="Joystick 1") -> ("JoystickDevRef"=w42:T1)  [unwired: 9 in, 1 out]
  n224 = call <vilib>:"WPI_JoystickRefNum Registry Get.vi"("refnum name"="Joystick 0") -> ("JoystickDevRef"=w46:T1)  [unwired: 1 in, 9 out]
  n225 = call <vilib>:"WPI_RobotDriveRefNum Registry Get.vi"("error in (no error)"="error in", "refnum name"="Left and Right Motors") -> ("RobotDriveDevRef"=w45:T17)  [unwired: 9 out]
  n226 = Bundle("JoystickDevRef"=w42, "JoystickDevRef"=w46, "RobotDriveDevRef"=w45) -> (w44:T18)  [unwired: 1 out]
  n227 = while {
    shift-right: [w629] -> _
    shift-left: w44 -> [w629]
    stop <- FALSE stop-if-true
    # "10 ms tasks go here"
    n228 = Wait (ms)(milliseconds to wait=u32 10) -> ()  [unwired: 1 out]
  }
  n229 = while {
    shift-right: [w632] -> _
    shift-left: w44 -> [w632]
    stop <- FALSE stop-if-true
    # "150 ms tasks go here"
    n230 = Wait (ms)(milliseconds to wait=u32 150) -> ()  [unwired: 1 out]
  }
